vi "AutoTrace Gauss Fit.vi"(8 "Line Counts":dbl[](array[numeric]), 11 "Line Position":dbl[](array[numeric])) -> (0 "Gauss fit error":dbl=0.06729316825119826, 2 "Gauss center":dbl, 3 "Gauss Width":dbl=1.5825811679814226 caption="standard deviation")   [LabVIEW 2020]
uses:
  <vilib>/Analysis/baseanly.llb/Mean (DBL).vi
  <vilib>/Analysis/3filter.llb/Butterworth Filter (DBL).vi
  <vilib>/Analysis/NI_AALPro.lvlib
  <vilib>/Analysis/NI_AALBase.lvlib
panel:
  out "NV location":dbl
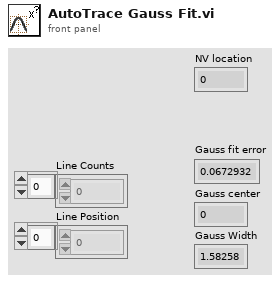
[diagram p1: front panel]
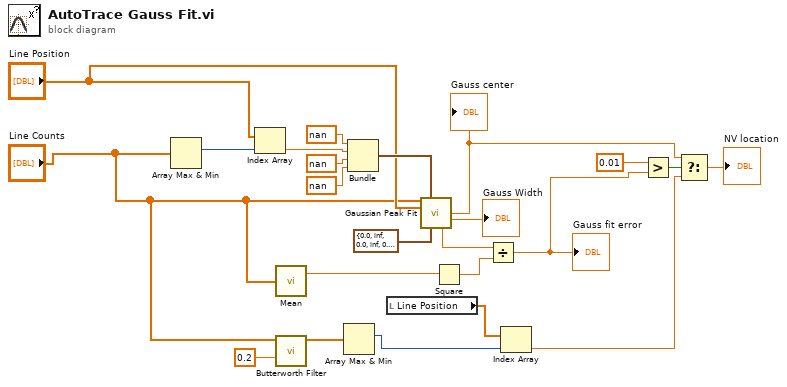
[diagram p0: block diagram]
diagram:
  n1 = Array Max & Min(array="Line Counts") -> (max index (indices)=w23:i32)  [unwired: 3 out]
  n2 = Index Array(array="Line Position", index=w23) -> (element=w20:dbl)
  n3 = call-poly <vilib>:"Mean.vi"("X"="Line Counts") -> ("mean"=w14:dbl)  [unwired: 1 out]
  n4 = call-poly <vilib>:"Butterworth Filter.vi"("high cutoff freq: fh"=0.2, "X"="Line Counts") -> ("Filtered X"=w9:dbl[])  [unwired: 6 in, 1 out]
  n5 = Array Max & Min(array=w9) -> (max index (indices)=w8:i32)  [unwired: 3 out]
  n6 = Bundle(nan, "Numeric"=w20, nan, nan) -> (w18:cluster{dbl, "Numeric":dbl, dbl, dbl})  [unwired: 1 in]
  n7 = local read "Line Position"() -> (w7:dbl[])
  n8 = call <vilib>:"Gaussian Peak Fit.vi"("Y"="Line Counts", "initial guess"=w18, "X"="Line Position", "parameter bounds"=cluster{dbl, dbl, dbl, dbl, dbl, dbl, dbl, dbl} {0.0, inf, 0.0, inf, 0.0, inf, 0.0, inf}) -> ("center"=w3:dbl, "standard deviation"=→"Gauss Width":dbl, "residue"=w13:dbl)  [unwired: 5 in, 4 out]
  "Gauss center" <- w3
  n9 = Square(x=w14) -> (x^2=w15:dbl)
  n10 = Divide(x=w13, y=w15) -> (x/y=w4:dbl)
  "Gauss fit error" <- w4
  n11 = Index Array(array=w7, index=w8) -> (element=w2:dbl)
  n12 = Greater?(x=0.01, y=w4) -> (0:w5:bool)
  n13 = Select(t=w3, s=w5, f=w2) -> (s? t:f=→"NV location":dbl)
